vi "Update motors target values.vi"(0 "Update Motors Notifier":refnum<notifier>, 1 "Right motor Clustered SDO":T1, 2 "Left motor Clustered SDO":T1, 3 "\"Pedals\" Status":T4 {"Acceleration pedal" scale=0.0..100.0 scale format="%#_6f%%"; "Break pedal" scale=0.0..100.0 scale format="%#_6f%%"}, 4 "Left Motor Status":T3, 5 "Right Motor Status":T3, 7 "Error Queue":refnum<queue>) -> (23 "Target Torque Left":i16(knob) scale=-1000.0..1000.0, 24 "Target Torque Right":i16(knob) scale=1000.0..-1000.0, 27 "Exit?":bool)   [LabVIEW 2016]
uses:
  RT/Pedals Status.ctl
  RT/Clustered SDO.ctl
  RT/Set target torque.vi
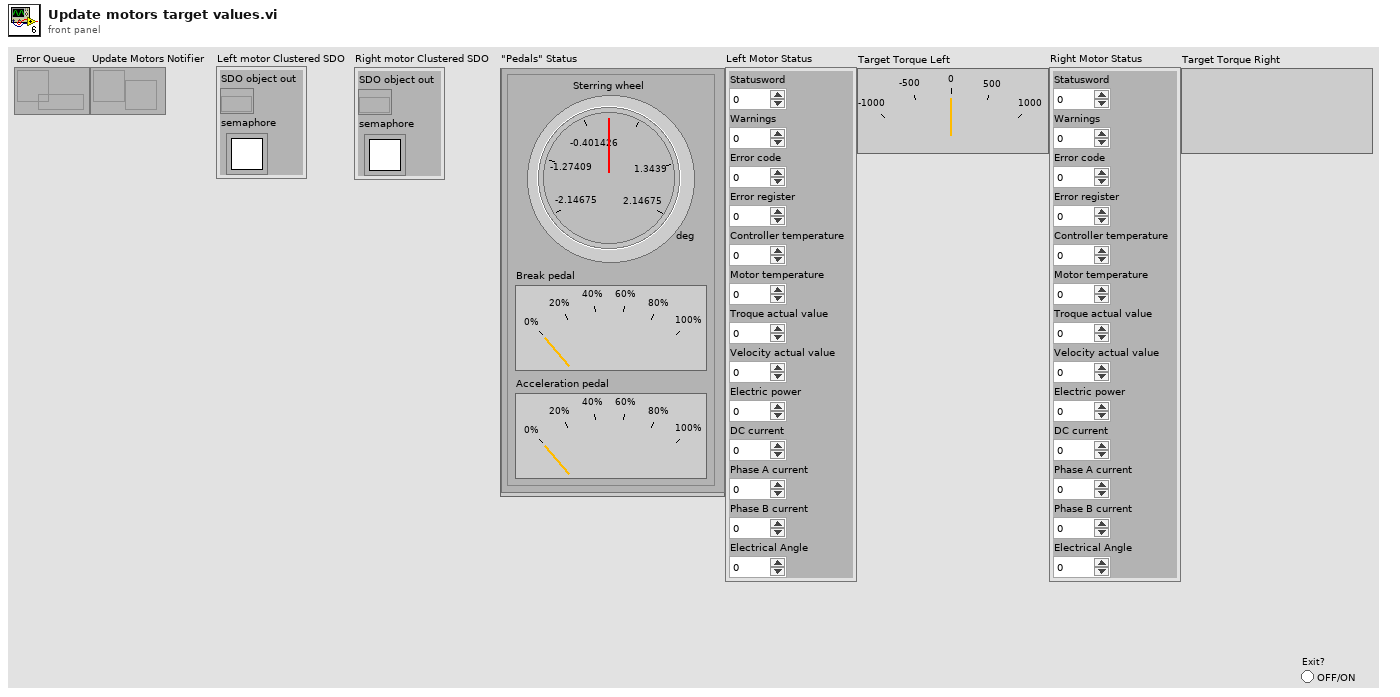
[diagram p1: front panel]
types:
  T1 = typedef "Clustered SDO.ctl" = cluster{"SDO object out":refnum<k20>, "semaphore":T2}
  T2 = typedef "Semaphore RefNum" = refnum<k1>
  T3 = cluster{"Statusword":u16, "Warnings":u16, "Error code":u16, "Error register":u8, "Controller temperature":u8, "Motor temperature":u8, "Troque actual value":i16, "Velocity actual value":i32, "Electric power":u32, "DC current":u32, "Phase A current":u16, "Phase B current":u16, "Electrical Angle":u16}
  T4 = typedef "Pedals Status.ctl" = cluster{"Acceleration pedal":dbl, "Break pedal":dbl, "Sterring wheel":dbl[unit]}
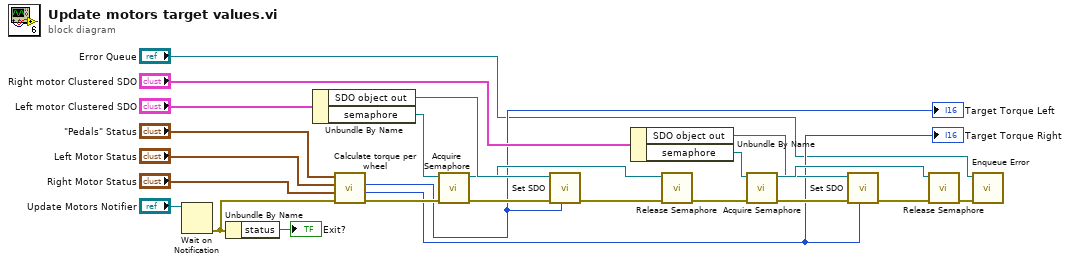
[diagram p0: block diagram]
diagram:
  n1 = Wait on Notification(notifier="Update Motors Notifier") -> (error out=w11:errorcluster)  [unwired: 3 in, 3 out]
  n2 = Unbundle By Name(w11) -> ("status"=→"Exit?":bool)
  n3 = Unbundle By Name("Left motor Clustered SDO") -> ("SDO object out"=w23:refnum<k20>, "semaphore"=w24:T2)
  n4 = call "Calculate torque per wheel.vi"("Error In"=w11, "Right Motor Status"="Right Motor Status", "Left Motor Status"="Left Motor Status", "\"Pedals\" Status"="\"Pedals\" Status") -> ("Error Out"=w22:errorcluster, "Target Torque Right"=w6:i16, "Target Torque Left"=w7:i16)  [unwired: 5 in]
  "Target Torque Left" <- w7
  "Target Torque Right" <- w6
  n5 = call <vilib>:"Acquire Semaphore.vi"("error in (no error)"=w22, "semaphore"=w24) -> ("error out"=w21:errorcluster, "semaphore out"=w19:T2)  [unwired: 3 in, 1 out]
  n6 = call-poly "Set SDO.vi"("Torque"=w7, "error in (no error)"=w21, "SDO object in"=w23) -> ("error out"=w20:errorcluster)  [unwired: 6 in, 2 out]
  n7 = Unbundle By Name("Right motor Clustered SDO") -> ("SDO object out"=w15:refnum<k20>, "semaphore"=w14:T2)
  n8 = call <vilib>:"Release Semaphore.vi"("error in (no error)"=w20, "semaphore"=w19) -> ("error out"=w13:errorcluster)  [unwired: 4 in, 1 out]
  n9 = call <vilib>:"Acquire Semaphore.vi"("error in (no error)"=w13, "semaphore"=w14) -> ("error out"=w16:errorcluster, "semaphore out"=w18:T2)  [unwired: 3 in, 1 out]
  n10 = call-poly "Set SDO.vi"("Torque"=w6, "error in (no error)"=w16, "SDO object in"=w15) -> ("error out"=w17:errorcluster)  [unwired: 6 in, 2 out]
  n11 = call <vilib>:"Release Semaphore.vi"("error in (no error)"=w17, "semaphore"=w18) -> ("error out"=w12:errorcluster)  [unwired: 4 in, 1 out]
  n12 = call "Enqueue Error.vi"("error in"=w12, "Error Queue"="Error Queue") -> ()  [unwired: 10 in]
